vi "Configure Broadcast Active.vi"(8 "error in (no error)":errorcluster, 10 "Active?":bool=TRUE, 11 "Debugger In":refnum<class "Debugger.lvclass">) -> (0 "error out":errorcluster, 3 "Debugger Out":refnum<class "Debugger.lvclass">)   [LabVIEW 2020]
uses:
  Debugger.lvclass
  C:/Users/anton/Documents/GitHub/triarc-debugger/source/Process/Debug Process.lvclass
  Process/Debug Process.lvclass/Debug Process.ctl
  Debugger.lvclass/Debugger.ctl
  <vilib>/Utility/error.llb/Clear Errors.vi
  <vilib>/Utility/error.llb/Error Cluster From Error Code.vi
  Process/Debug Process.lvclass
  C:/Users/anton/Documents/GitHub/triarc-debugger/source/Debugger/Debugger.lvclass
  C:/Users/anton/Documents/GitHub/triarc-debugger/source/Debug Data Event/Debug Data Listener.lvclass
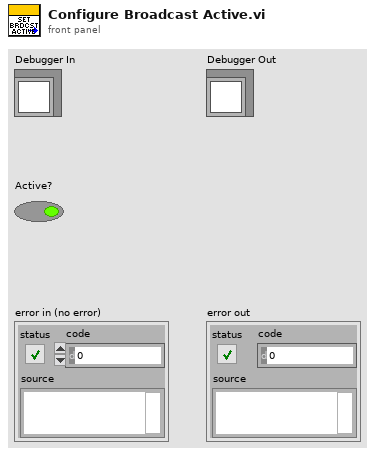
[diagram p1: front panel]
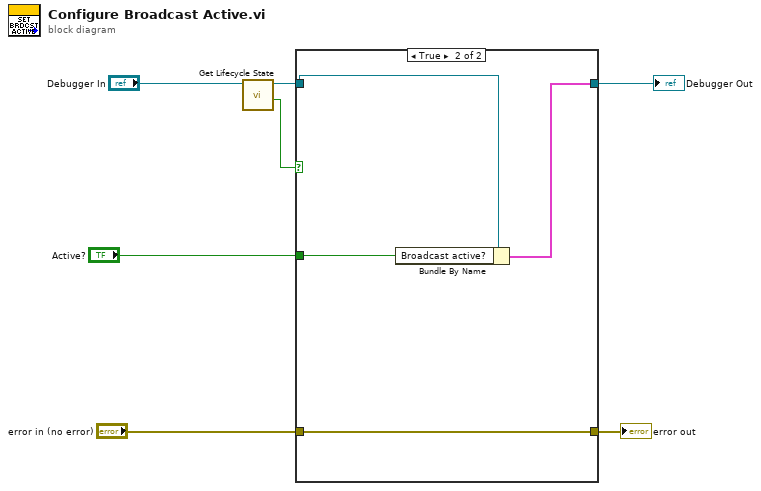
[diagram p0: block diagram]
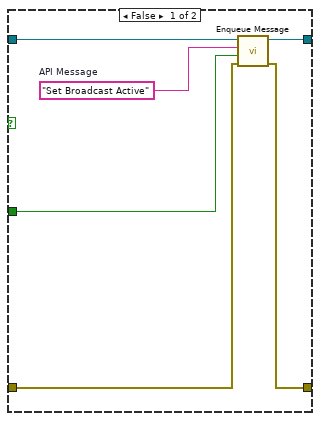
[diagram p2: hidden frame]
diagram:
  n1 = call "Get Lifecycle State.vi"("Process In"="Debugger In") -> ("In Process Loop?"=w1:bool, "Process Out"=w2:refnum<class "Debugger.lvclass">)  [unwired: 7 in, 2 out]
  n2 = case shown="True" w1 {
    tunnel: [w13 w16] -> w7
    tunnel: [w12 w14] -> w6
    tunnel: "error in (no error)" -> [w11 w14]
    tunnel: "Active?" -> [w9 w15]
    tunnel: w2 -> [w8 w17]
    frame False {
      w10 = "Set Broadcast Active"  # API Message
      n3 = call "Enqueue Message.vi"("error in (no error)"=w11, "Message Data"=w9, "Message"=w10, "Process In"=w8) -> ("error out"=w12:errorcluster, "Process Out"=w13:refnum<class "Debugger.lvclass">)  [unwired: 6 in]
    }
    frame True {
      n4 = Bundle By Name(cluster=w17, "Broadcast active?"=w15) -> (w16:cluster{})
    }
  }
  "error out" <- w6
  "Debugger Out" <- w7
